vi "MH_OTF_Subtraction_Buffers_Method.vi"(8 "ofl":u64, 9 "Buffer":u32[](array[numeric]), 10 "Cluster In":T1 {"Coincidence Window" format="%#_13g"; "Delay12" format="%#_13g"; "Delay02" format="%#_13g"; "Delay01" format="%#_13g"}, 11 "Buffer Length":i32=100) -> (0 "ofl out":u64, 2 "cluster Out":T1 {"Coincidence Window" format="%#_13g"; "Delay12" format="%#_13g"; "Delay02" format="%#_13g"; "Delay01" format="%#_13g"})   [LabVIEW 2023]
uses:
  Get_Delays_Ctrl.ctl
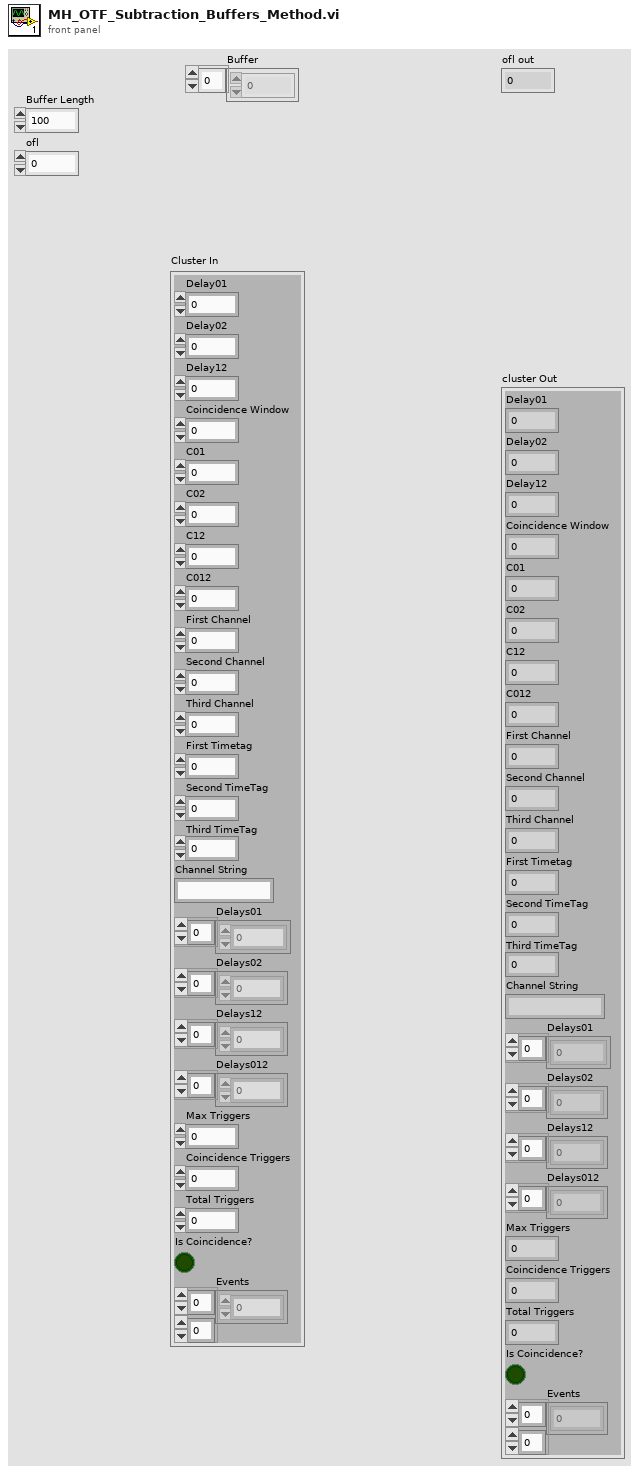
[diagram p1: front panel]
types:
  T1 = typedef "Get_Delays_Ctrl.ctl" = cluster{"Delay01":dbl, "Delay02":dbl, "Delay12":dbl, "Coincidence Window":dbl, "C01":u32, "C02":u32, "C12":u32, "C012":u32, "First Channel":dbl, "Second Channel":dbl, "Third Channel":dbl, "First Timetag":dbl, "Second TimeTag":dbl, "Third TimeTag":dbl, "Channel String":string, "Delays01":sgl[], "Delays02":dbl[], "Delays12":dbl[], "Delays012":dbl[], "Max Triggers":i32, "Coincidence Triggers":i32, "Total Triggers":i32, "Is Coincidence?":bool, "Events":u64[][]}
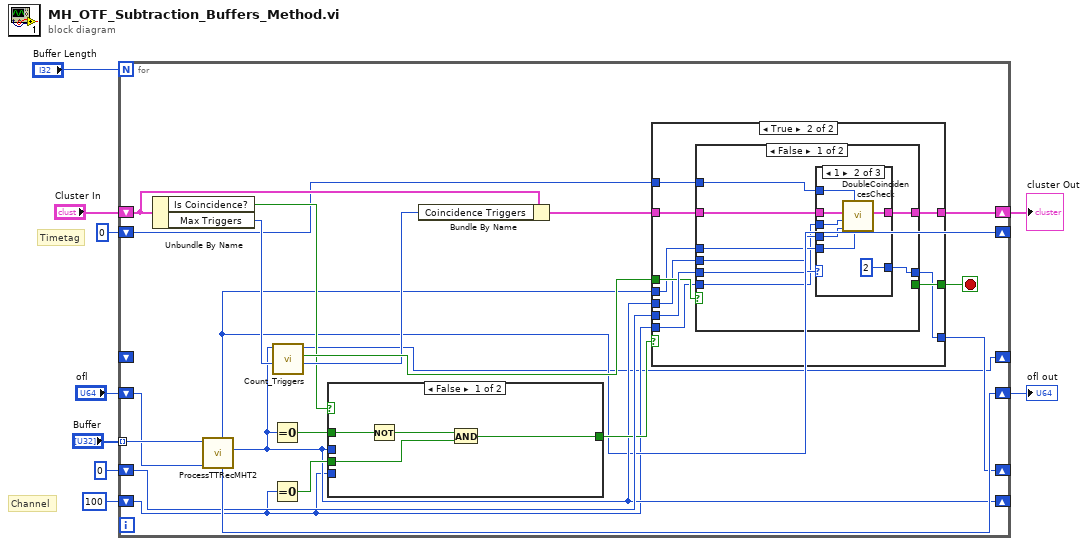
[diagram p0: block diagram]
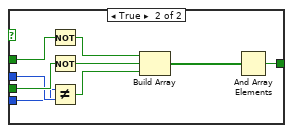
[diagram p2: hidden frame]
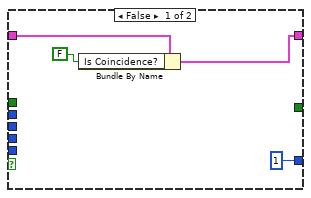
[diagram p3: hidden frame]
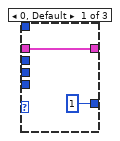
[diagram p4: hidden frame]
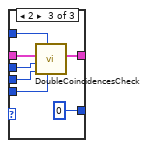
[diagram p5: hidden frame]
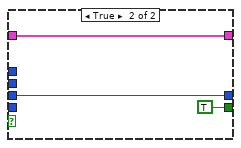
[diagram p6: hidden frame]
diagram:
  # "Channel"
  # "Timetag"
  n1 = for {
    N: "Buffer Length" -> [_]
    shift-right: [w30] -> w1
    shift-left: "Cluster In" -> [w26]
    tunnel: "Buffer" -> [w29] mode=indexing
    shift-right: [w27] -> w7
    shift-left: "ofl" -> [w28]
    shift-right: [w14] -> _
    shift-left: u32 100 ("channel") -> [w12]
    shift-right: [w20] -> _
    shift-left: u32 0 ("channel") -> [w21]
    shift-right: [w13] -> _
    shift-left: u64 0 ("timetag") -> [w11]
    shift-right: [w10] -> _
    shift-left: _ -> [_]
    stop <- w15 stop-if-true
    n2 = Unbundle By Name(w26) -> ("Is Coincidence?"=w19:bool, "Max Triggers"=w24:i32)
    n3 = call "ProcessTTRecMHT2.vi"("oflcorr_in"=w28, "rawbits"=w29) -> ("channel"=w14:u32, "oflcorr_out"=w27:u64, "timetag"=w13:u64)  [unwired: 4 in, 3 out]
    n4 = Equal To 0?(x=w14) -> (x = 0?=w16:bool)
    n5 = Equal To 0?(x=w12) -> (x = 0?=w17:bool)
    n6 = call "Count_Triggers.vi"("Max Triggers"=w24, "channel"=w14) -> ("Coincidence Triggers"=w23:u64, "Max triggers?"=w25:bool, "Total Triggers Out"=w10:u64)  [unwired: 7 in]
    n7 = case shown="False" w19 {
      tunnel: [w31 w35] -> w18
      tunnel: w17 -> [w32 w42]
      tunnel: w16 -> [w34 w43]
      tunnel: w14 -> [_ w41]
      tunnel: w12 -> [_ w40]
      frame False {
        n8 = Not(x=w34) -> (.not. x?=w33:bool)
        n9 = And(x=w33, y=w32) -> (x .and. y?=w31:bool)
      }
      frame True {
        n10 = Not(x=w43) -> (.not. x?=w39:bool)
        n11 = Not(x=w42) -> (.not. x?=w38:bool)
        n12 = Not Equal?(x=w40, y=w41) -> (x != y?=w37:bool)
        n13 = Build Array(w39, w38, w37) -> (w36:bool[])
        n14 = And Array Elements(Boolean array=w36) -> (logical AND=w35:bool)
      }
    }
    n15 = Bundle By Name(cluster=w26, "Coincidence Triggers"=w23) -> (w22:T1)
    n16 = case shown="True" w18 {
      tunnel: [w45 w57] -> w30
      tunnel: w21 -> [_ w56]
      tunnel: w25 -> [_ w55]
      tunnel: w22 -> [w46 w54]
      tunnel: [u32 1 ("channel") w52] -> w20
      tunnel: [_ w53] -> w15
      tunnel: w14 -> [_ w51]
      tunnel: w13 -> [_ w50]
      tunnel: w12 -> [_ w49]
      tunnel: w11 -> [_ w48]
      frame False {
        n17 = Bundle By Name(cluster=w46, "Is Coincidence?"=FALSE) -> (w45:T1)
      }
      frame True {
        n18 = case shown="False" w55 {
          tunnel: [w65 w84] -> w57
          tunnel: w56 -> [w64 w83]
          tunnel: w54 -> [w63 w84]
          tunnel: [w62 w83] -> w52
          tunnel: [_ TRUE] -> w53
          tunnel: w51 -> [w61 _]
          tunnel: w50 -> [w60 _]
          tunnel: w49 -> [w59 _]
          tunnel: w48 -> [w58 _]
          frame False {
            n19 = case shown="1" w64 {
              tunnel: w63 -> [w67 w74 w79]
              tunnel: [w67 w73 w81] -> w65
              tunnel: [u32 1 ("channel") u32 2 ("channel") u32 0 ("channel")] -> w62
              tunnel: w61 -> [_ w71 w77]
              tunnel: w60 -> [_ w70 w78]
              tunnel: w59 -> [_ w69 w76]
              tunnel: w58 -> [_ w68 w75]
              frame 0, Default {
              }
              frame 1 {
                n20 = call "DoubleCoincidencesCheck.vi"("Time B"=w70, "Time A"=w68, "ChB"=w71, "ChA"=w69, "Cluster In"=w74) -> ("cluster Out"=w73:T1)  [unwired: 6 in]
              }
              frame 2 {
                n21 = call "DoubleCoincidencesCheck.vi"("Time B"=w78, "Time A"=w75, "ChB"=w77, "ChA"=w76, "Cluster In"=w79) -> ("cluster Out"=w81:T1)  [unwired: 6 in]
              }
            }
          }
          frame True {
          }
        }
      }
    }
  }
  "ofl out" <- w7
  "cluster Out" <- w1
